vi "TestCloneAPI.vi"() -> ()   [LabVIEW 2018, in "SyncModule.lvlib"]
uses:
  SyncModule.lvlib
  SyncPlugins/SyncPluginBase/Typedefs/clTimedTrigger.ctl
  SyncPlugins/PXI_MultiTrig/Typedefs/clClocks.ctl
  TestInfo.ctl
  <userlib>/NIST/ModuleAdminLib/CloneRegistration/CloneRegistration.lvclass
  <userlib>/NIST/ModuleAdminLib/ModuleAdmin/ModuleAdmin.lvclass/ModuleAdmin.ctl
  <userlib>/NIST/ModuleAdminLib/ModuleAdmin/ModuleAdmin.lvclass
  PublicAPI/Arguments/Broadcasts/clDidInit.ctl
  PublicAPI/Arguments/Requests/clStopArgument.ctl
  <vilib>/Utility/error.llb/DialogType.ctl
  <userlib>/NIST/ModuleAdminLib/ModuleAdmin/Accessors/Read CloneRegRef.vi
  <userlib>/NIST/ModuleAdminLib/ModuleAdmin/Accessors/Write CloneRegRef.vi
  SyncPlugins/SyncPluginBase/SyncPluginBase.lvclass
  SyncPlugins/PXI_MultiTrig/PXI_MultiTrig.lvclass
panel:
  in  "btnSetClkProperties":bool
  in  "ClockProperties":T1[](array[typedef])
  in  "btnClkProperties":bool
  in  "Parameters":string="PXI_Trig2"
  out "Info":string[](array[string])
  in  "btnGetInfo":bool
  in  "Timed Trigger":T2={"TriggerName"="Timed_1", "Time after next UTC Second"=0.1, "Trigger Duration"=0.1, "Edge"=enum."Rising"}
  in  "btnTimedTrig":bool
  in  "btnSoftwareTrig":bool
  in  "btnPref":bool
  out "Locked?":bool
  in  "btnRequestLockStatus":bool
  out "TriggerTime":timestamp format="%^<%.3X\n%x>T"
  in  "btnRequestTriggerTime":bool
  in  "Show Panel":bool=TRUE
  in  "Plugin Type":u16(ring) items=["Local", "NI PXI 6682", "Debug Sync IOP", "6683H class Dyn3", "AbsPhase", "SaveWaveform", "Dyn3 PMU Cal", "HIL_Sync", "Offset Digi Trigger", "PMU Cal Cal"]
  in  "btnLoadPlugin":bool
  out "Path":path
  in  "btnRequestINIPath":bool
  in  "btnRemove":bool
  out "Status Log":string
  out "Active Modules (Array)":string[](array[string])
  in  "btnAdd":bool
  in  "btnStop":bool
  in  "Select Module":i32(ring)=-1 caption="Select Module to send Request" items=["All"=-1, "4140002"=4140002]
  # "Hidden"
  # "Visible"
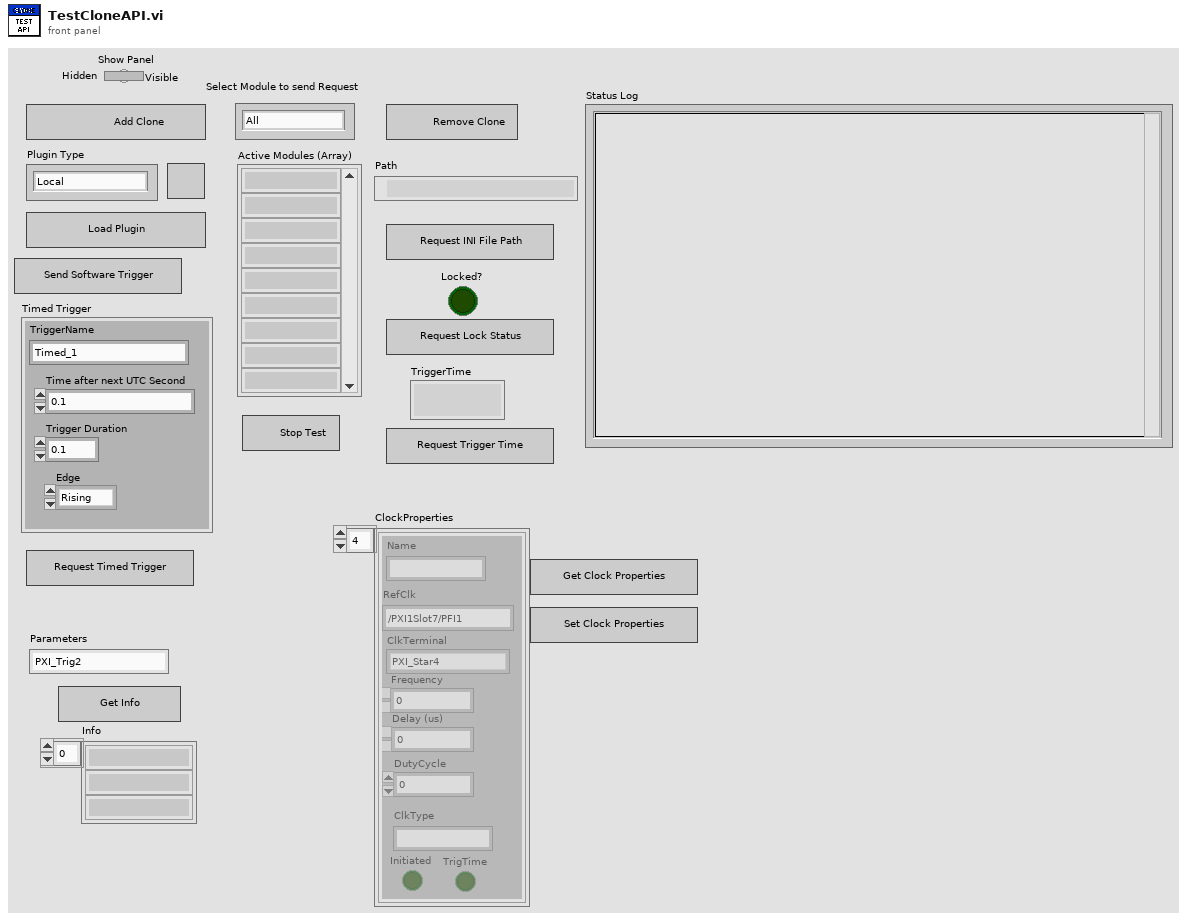
[diagram p1: front panel]
types:
  T1 = typedef "SyncPlugins.lvlib/PXI_MultiTrig.lvclass/clClocks.ctl" = cluster{"Name":string, "RefClk":string, "ClkTerminal":string, "Frequency":dbl, "DutyCycle":dbl, "ClkType":string, "Initiated":bool, "TrigTime":bool, "Delay":dbl}
  T2 = typedef "SyncPlugins.lvlib/SyncPluginBase.lvclass/clTimedTrigger.ctl" = cluster{"TriggerName":string, "Time after next UTC Second":dbl, "Trigger Duration":dbl, "Edge":enum16{"Rising", "Falling"}}
  T3 = typedef "SyncModule.lvlib/TestInfo.ctl" = cluster{"PluginIniFilePaths":path[]}
  T4 = typedef "SyncModule.lvlib/clBroadcastEvents.ctl" = cluster{"DidInit":refnum<user-event>, "StatusUpdate":refnum<user-event>, "ErrorReport":refnum<user-event>, "DidStop":refnum<user-event>, "PathToINI":refnum<user-event>, "TriggerTime":refnum<user-event>, "LockStatus":refnum<user-event>, "Info":refnum<user-event>, "ClockProperties":refnum<user-event>}
  T5 = typedef "SyncModule.lvlib/clDidInit.ctl" = cluster{"Init?":bool, "ModuleAdmin":refnum<class "ModuleAdmin.lvclass">}
  T6 = typedef "SyncModule.lvlib/clStopArgument.ctl" = cluster{"Exit via Stop Module Req?":bool, "Wait for Module to stop?":bool, "ModuleAdmin":refnum<class "ModuleAdmin.lvclass">}
  T7 = typedef "DialogType.ctl" = u16
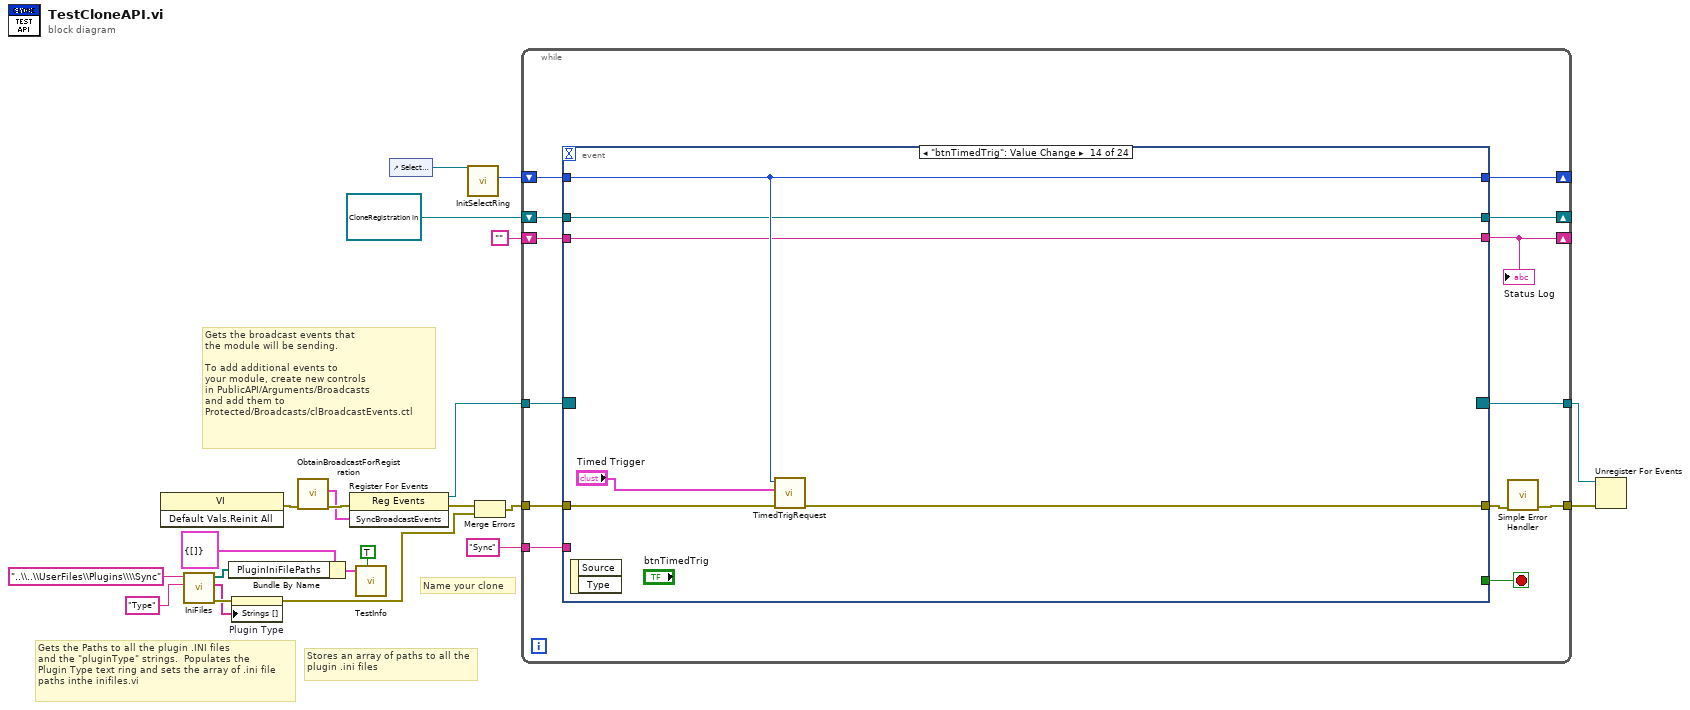
[diagram p0: block diagram]
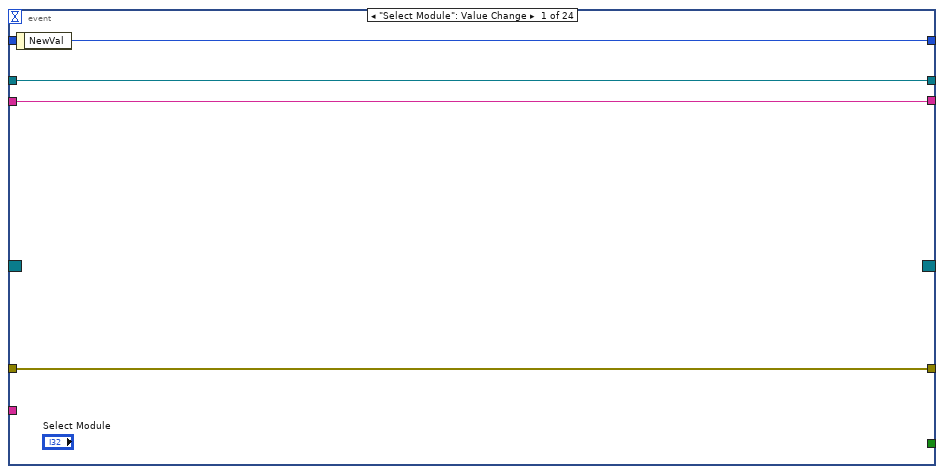
[diagram p2: hidden frame]
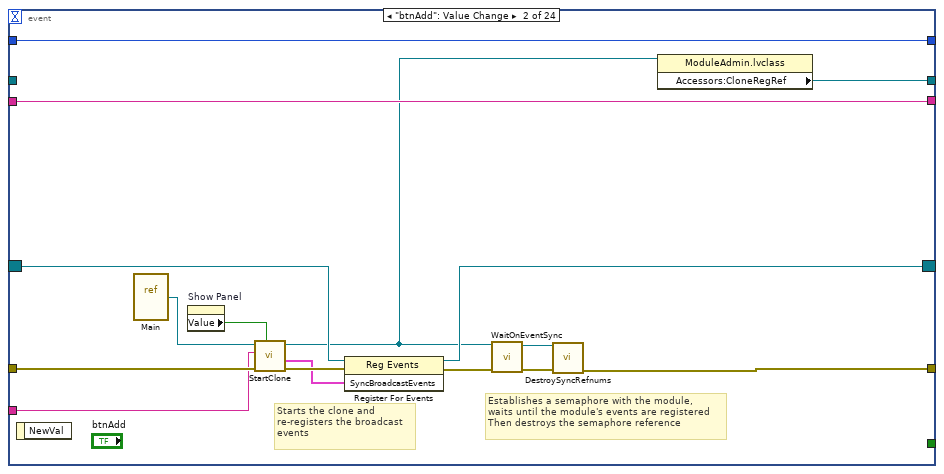
[diagram p3: hidden frame]
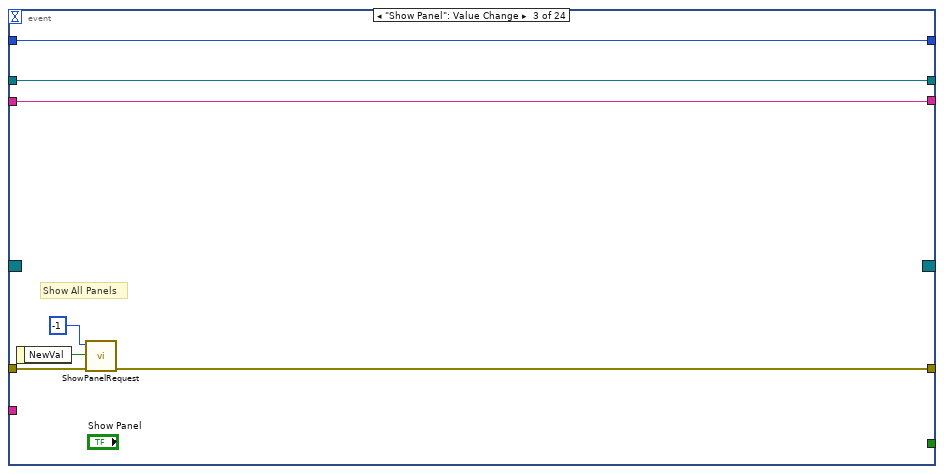
[diagram p4: hidden frame]
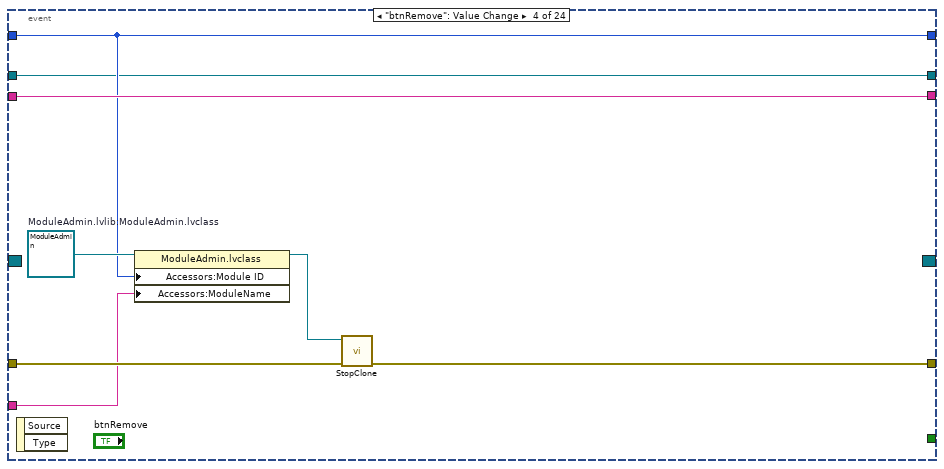
[diagram p5: hidden frame]
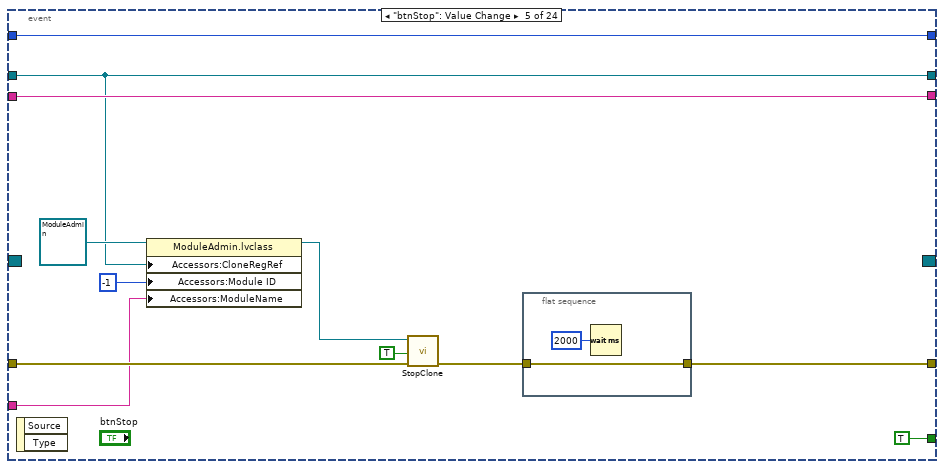
[diagram p6: hidden frame]
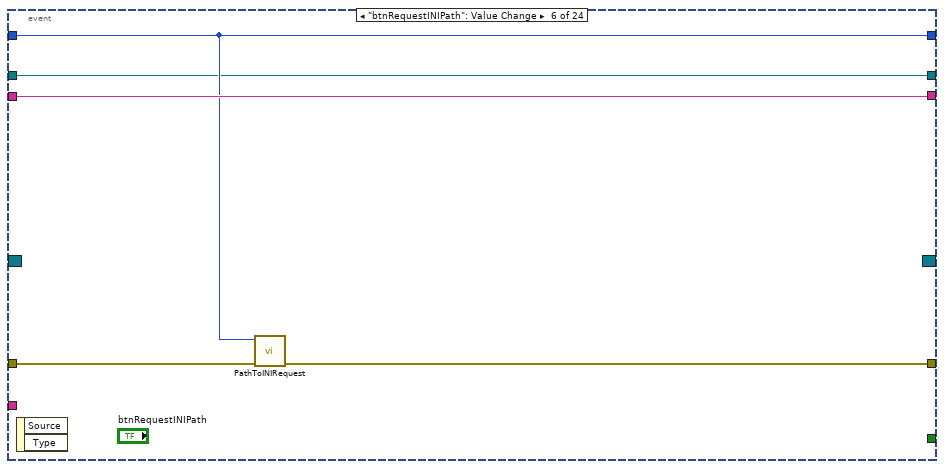
[diagram p7: hidden frame]
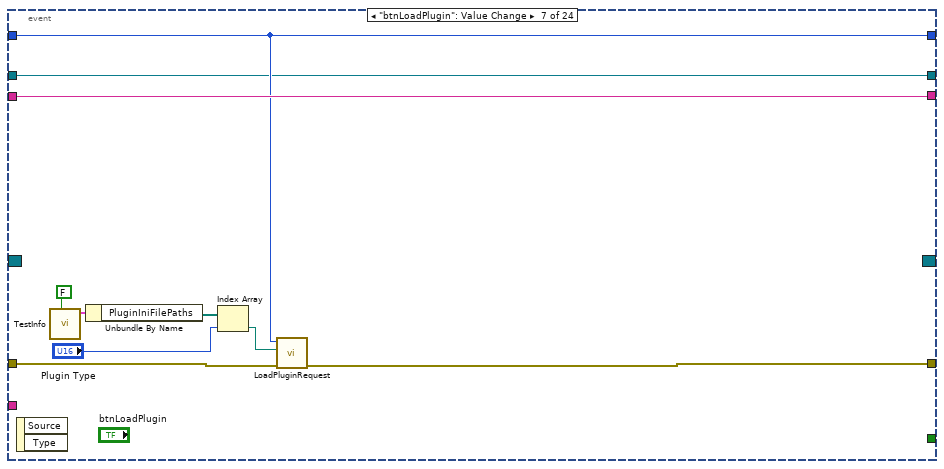
[diagram p8: hidden frame]
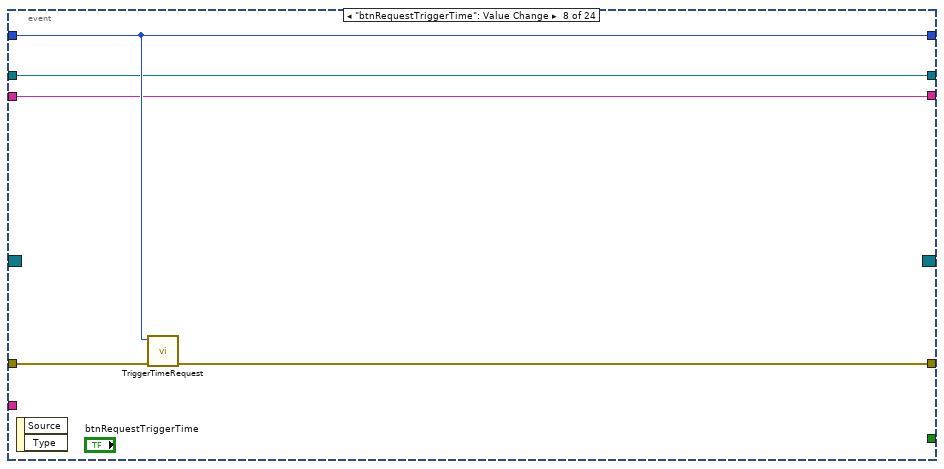
[diagram p9: hidden frame]
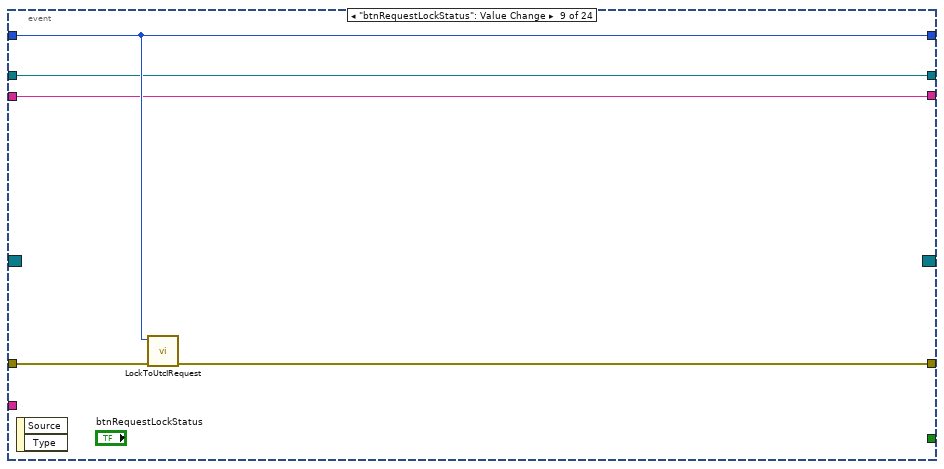
[diagram p10: hidden frame]
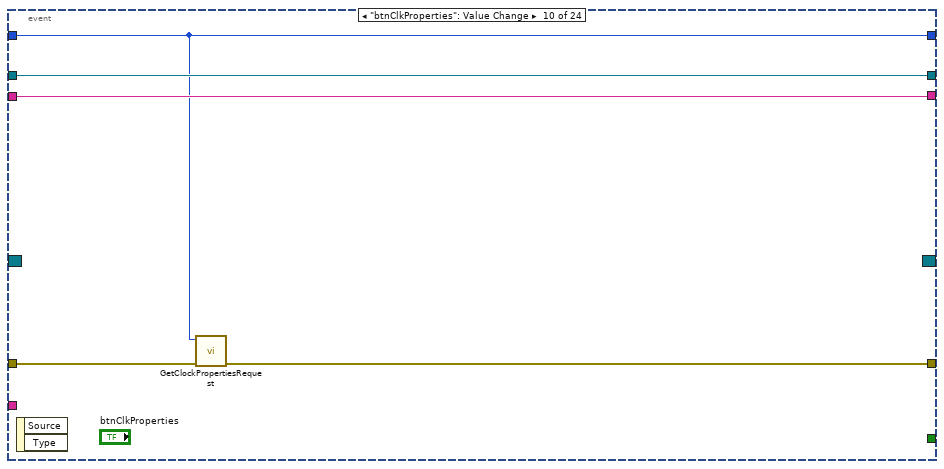
[diagram p11: hidden frame]
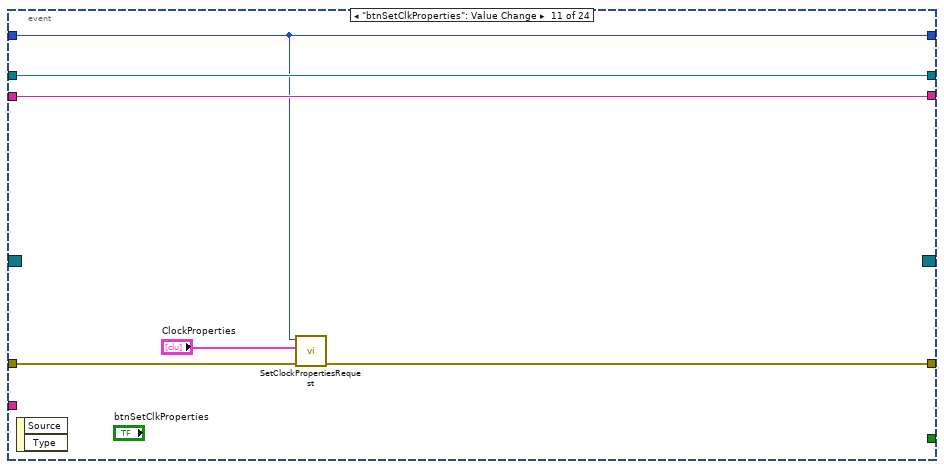
[diagram p12: hidden frame]
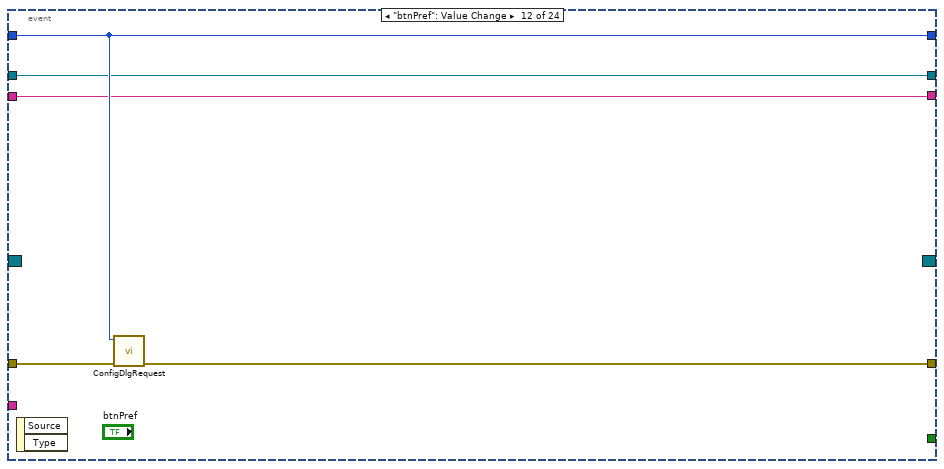
[diagram p13: hidden frame]
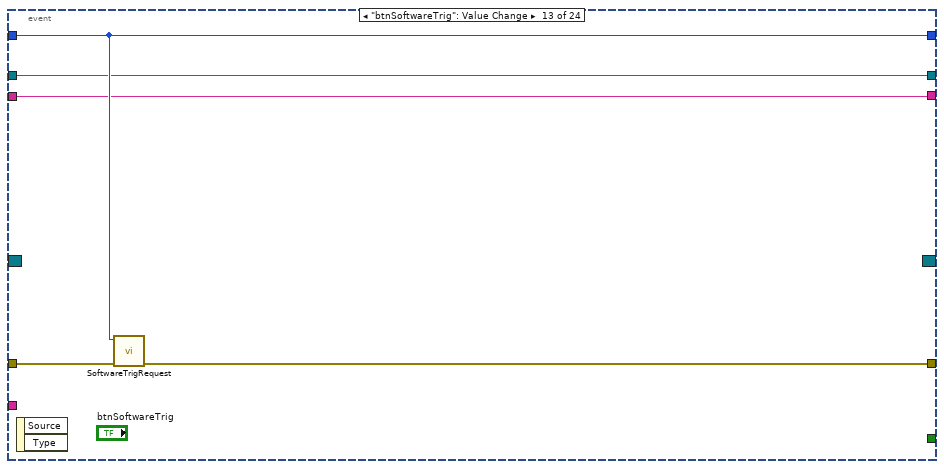
[diagram p14: hidden frame]
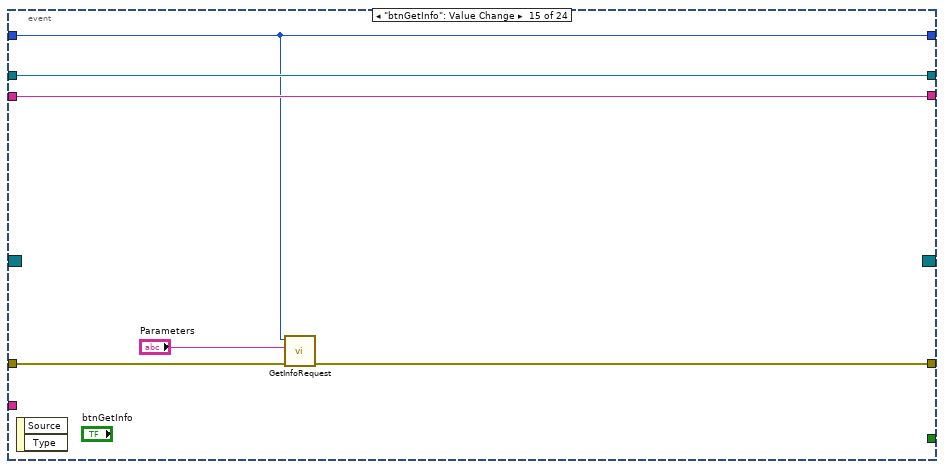
[diagram p15: hidden frame]
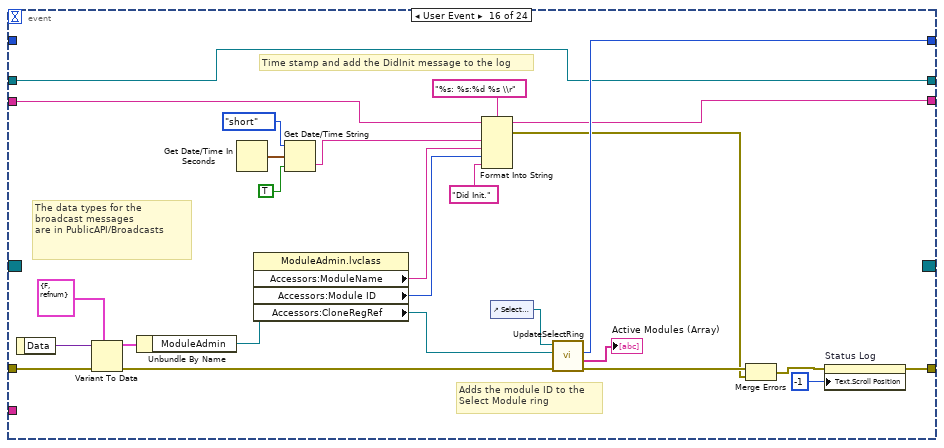
[diagram p16: hidden frame]
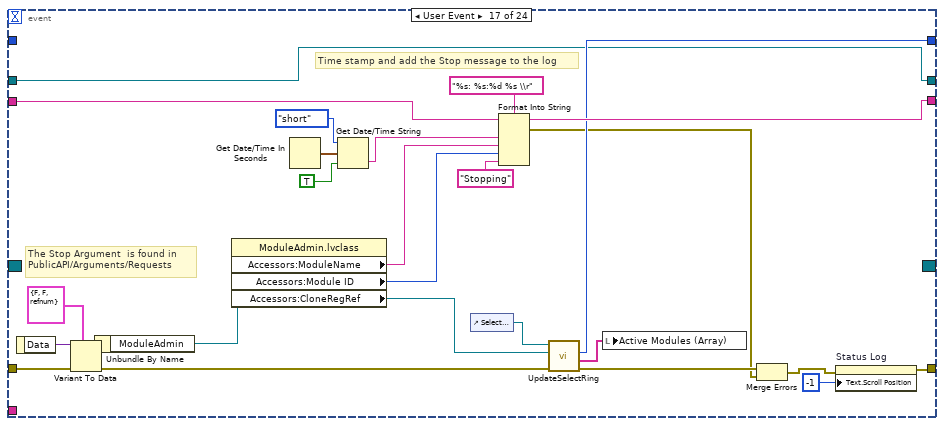
[diagram p17: hidden frame]
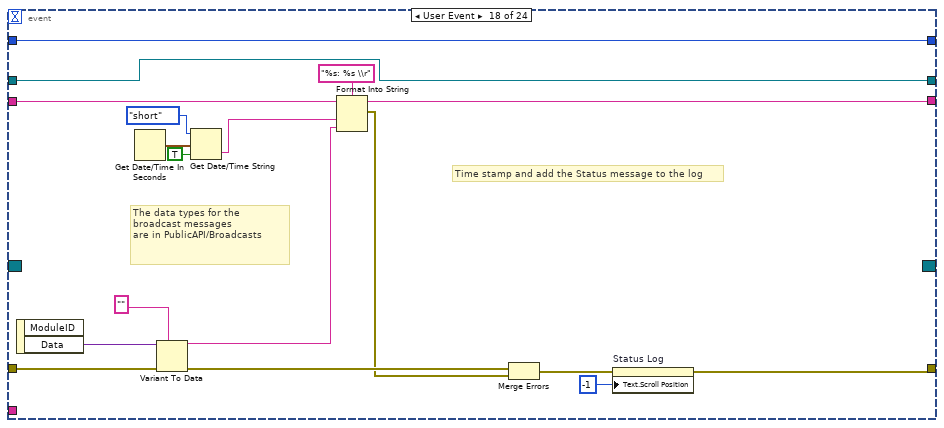
[diagram p18: hidden frame]
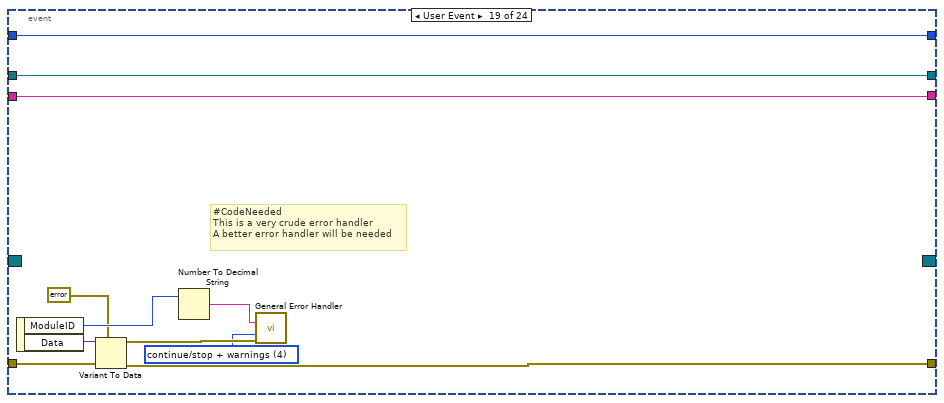
[diagram p19: hidden frame]
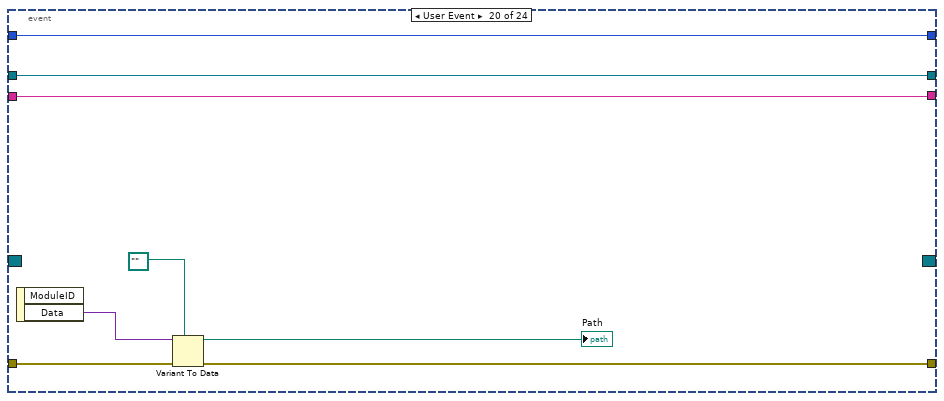
[diagram p20: hidden frame]
diagram:
  # "Stores an array of paths to all the plugin .ini files"
  # "Gets the Paths to all the plugin .INI files\nand the \"pluginType\" strings.  Populates the \nPlugin Type text ring and sets the array of .ini file\npaths inthe inifiles.vi"
  # "Name your clone"
  # "Gets the broadcast events that\nthe module will be sending.\n\nTo add additional events to\nyour module, create new controls\nin PublicAPI/Arguments/Broadcasts\nand add them to\nProtected/Broadcasts/clBroadcastEvents.ctl"
  n1 = invoke class="VI" method="Default Vals.Reinit All"() -> (error out=w20:errorcluster)  [unwired: 3 in, 2 out]
  n2 = call "IniFiles.vi"("iniKey"="Type", "name or relative path"="..\\..\\UserFiles\\Plugins\\\\Sync") -> ("error out"=w13:errorcluster, "Types"=w12:string[], "IniFilePaths"=w11:path[])  [unwired: 7 in]
  n3 = Bundle By Name(cluster=T3 {"PluginIniFilePaths"=[]} ("TestInfo"), "PluginIniFilePaths"=w11) -> (w10:T3)
  n4 = property on="Plugin Type" class="Ring (strict)"(error in=w13, "Strings []"=w12) -> (error out=w7:errorcluster)  [unwired: 1 in, 1 out]
  n5 = call "ObtainBroadcastForRegistration.vi"("error in (no error)"=w20) -> ("error out"=w19:errorcluster, "SyncBroadcastEvents"=w18:T4)  [unwired: 9 in]
  n6 = register-events(error in=w19, w18) -> (reference out=w16:refnum<event-registration>, error out=w17:errorcluster)  [unwired: 1 in]
  n7 = call "TestInfo.vi"("Set (f)"=TRUE, "TestInfo 2"=w10) -> ()  [unwired: 9 in, 1 out]
  n8 = control-ref of="Select Module"() -> (w22:refnum<vi>)
  n9 = call "InitSelectRing.vi"("Ring Refnum"=w22) -> ("Module Ring Value"=w21:i32)  [unwired: 9 in, 1 out]
  n10 = Merge Errors(w17, w7) -> (w8:errorcluster)
  n11 = while {
    shift-right: [w35] -> _
    shift-left: w21 -> [w26]
    tunnel: w8 -> [w33]
    tunnel: w16 -> [w30]
    tunnel: [w31] -> w3
    shift-right: [w29] -> _
    shift-left: "" -> [w28]
    tunnel: "Sync" ("ModuleName") -> [w27]
    tunnel: [w25] -> w2
    shift-right: [w24] -> _
    shift-left: refnum<data-value> refnum ("Accessors:CloneRegRef") -> [w23]
    stop <- w34 stop-if-true
    n12 = event shown="[13] \"btnTimedTrig\": Value Change" {
      selector: w30 -> [_ w47 _ _ _ _ _ _ _ _ _ _ _ _ _ _ _ _ _ _ _ _ _ _]
      dyn-events: [_ w46 _ _ _ _ _ _ _ _ _ _ _ _ _ _ _ _ _ _ _ _ _ _] -> w25
      timeout: _ -> [_ _ _ _ _ _ _ _ _ _ _ _ _ _ _ _ _ _ _ _ _ _ _ _]
      tunnel: w26 -> [_ w55 w58 w66 w82 w88 w96 w103 w108 w111 w116 w124 w129 w135 w138 _ _ w212 w218 w230 w243 w251 w255 w264]
      tunnel: [w39 w55 w58 w66 w82 w88 w96 w103 w108 w111 w116 w124 w129 w135 w138 w163 w181 w212 w218 w230 w243 w251 w255 w264] -> w35
      tunnel: [_ _ _ _ TRUE _ _ _ _ _ _ _ _ _ _ _ _ _ _ _ _ _ _ _] -> w34
      tunnel: w33 -> [w37 w54 w61 w69 w80 w87 w98 w104 w109 w114 w120 w125 w130 w136 w142 w168 w190 w209 w222 w226 w246 w254 w262 w268]
      tunnel: [w37 w48 w59 w68 w71 w86 w97 w101 w106 w110 w119 w121 w126 w132 w137 w144 w170 w197 w221 w225 w233 w252 w258 w267] -> w32
      tunnel: [w38 w44 w57 w70 w78 w89 w99 w102 w107 w113 w118 w123 w128 w134 w140 w156 w187 w206 w217 w231 w240 w250 w257 w266] -> w29
      tunnel: w28 -> [w38 w44 w57 w70 w78 w89 w99 w102 w107 w113 w118 w123 w128 w134 w140 w155 w188 w211 w217 w231 w241 w250 w257 w266]
      tunnel: w27 -> [_ w43 _ w65 w76 _ _ _ _ _ _ _ _ _ _ _ _ _ _ _ _ _ _ _]
      tunnel: [w36 w40 w56 w63 w73 w85 w90 w100 w105 w112 w117 w122 w127 w133 w139 w146 w172 w199 w214 w224 w235 w247 w256 w265] -> w24
      tunnel: w23 -> [w36 _ w56 w63 w73 w85 w90 w100 w105 w112 w117 w122 w127 w133 w139 w146 w172 w199 w214 w224 w235 w247 w256 w265]
      event "Select Module": Value Change {
        n13 = event-data() -> ("NewVal"=w39:i32)  [unwired: 1 in]
      }
      event "btnAdd": Value Change {
        # "Establishes a semaphore with the module,\nwaits until the module's events are registered\nThen destroys the semaphore reference"
        # "Starts the clone and\nre-registers the broadcast \nevents"
        n14 = event-data() -> ()  [unwired: 1 in, 1 out]
        n15 = vi-ref "Main.vi"() -> (w45:refnum<vi>)
        n16 = property on="Show Panel" class="Bool (strict)"() -> ("Value"=w42:bool)  [unwired: 2 in, 2 out]
        n17 = call "StartClone.vi"("ShowPanel? (f)"=w42, "error in (no error)"=w54, "ModuleName"=w43, "VI Refnum"=w45) -> ("error out"=w53:errorcluster, "SyncBroadcastEvents"=w49:T4, "ModuleAdmin"=w41:refnum<class "ModuleAdmin.lvclass">)  [unwired: 5 in]
        n18 = register-events(reference=w47, error in=w53, w49) -> (reference out=w46:refnum<event-registration>, error out=w52:errorcluster)
        n19 = call <userlib>:"WaitOnEventSync.vi"("error in (no error)"=w52, "ModuleAdmin"=w41) -> ("error out"=w51:errorcluster, "ModuleAdmin"=w50:refnum<class "ModuleAdmin.lvclass">)  [unwired: 8 in]
        n20 = call <userlib>:"DestroySyncRefnums.vi"("error in (no error)"=w51, "ModuleAdmin"=w50) -> ("error out"=w48:errorcluster)  [unwired: 9 in]
        n21 = property class="ModuleAdmin.lvclass"(reference=w41) -> ("Accessors:CloneRegRef"=w40:refnum<data-value>)  [unwired: 1 in, 2 out]
      }
      event "Show Panel": Value Change {
        # "Show All Panels"
        n22 = event-data() -> ("NewVal"=w62:bool)  [unwired: 1 in]
        n23 = call "ShowPanelRequest.vi"("error in (no error)"=w61, "ShowPanel?"=w62, "ModuleID"=-1) -> ("error out"=w59:errorcluster)  [unwired: 8 in]
      }
      event "btnRemove": Value Change {
        w67 = refnum<class "ModuleAdmin.lvclass"> refnum  # ModuleAdmin.lvlib:ModuleAdmin.lvclass
        n24 = event-data() -> ()  [unwired: 1 in, 2 out]
        n25 = property class="ModuleAdmin.lvclass"(reference=w67, "Accessors:Module ID"=w66, "Accessors:ModuleName"=w65) -> (reference out=w64:refnum<class "ModuleAdmin.lvclass">)  [unwired: 1 in, 1 out]
        n26 = call "StopClone.vi"("error in (no error)"=w69, "ModuleAdmin"=w64) -> ("error out"=w68:errorcluster)  [unwired: 9 in]
      }
      event "btnStop": Value Change {
        n27 = event-data() -> ()  [unwired: 1 in, 2 out]
        n28 = property class="ModuleAdmin.lvclass"(reference=refnum<class "ModuleAdmin.lvclass"> refnum ("ModuleAdmin.lvlib:ModuleAdmin.lvclass"), "Accessors:CloneRegRef"=w73, "Accessors:Module ID"=-1 ("Module ID"), "Accessors:ModuleName"=w76) -> (reference out=w75:refnum<class "ModuleAdmin.lvclass">)  [unwired: 1 in, 1 out]
        n29 = call "StopClone.vi"("error in (no error)"=w80, "Wait for Module to stop?"=TRUE, "ModuleAdmin"=w75) -> ("error out"=w72:errorcluster)  [unwired: 8 in]
        n30 = flat-sequence {
          tunnel: w72 -> [w83]
          tunnel: [w83] -> w71
          frame #0 {
            n31 = Wait (ms)(milliseconds to wait=u32 2000) -> ()  [unwired: 1 out]
          }
        }
      }
      event "btnRequestINIPath": Value Change {
        n32 = event-data() -> ()  [unwired: 1 in, 2 out]
        n33 = call "PathToINIRequest.vi"("error in (no error)"=w87, "ModuleID"=w88) -> ("error out"=w86:errorcluster)  [unwired: 9 in]
      }
      event "btnLoadPlugin": Value Change {
        n34 = event-data() -> ()  [unwired: 1 in, 2 out]
        n35 = call "TestInfo.vi"("Set (f)"=FALSE) -> ("TestInfo"=w94:T3)  [unwired: 10 in]
        n36 = Unbundle By Name(w94) -> ("PluginIniFilePaths"=w93:path[])
        n37 = Index Array(array=w93, index="Plugin Type") -> (element=w91:path)
        n38 = call "LoadPluginRequest.vi"("error in (no error)"=w98, "PathToPluginINI"=w91, "ModuleID"=w96) -> ("error out"=w97:errorcluster)  [unwired: 8 in]
      }
      event "btnRequestTriggerTime": Value Change {
        n39 = event-data() -> ()  [unwired: 1 in, 2 out]
        n40 = call "TriggerTimeRequest.vi"("error in (no error)"=w104, "ModuleID"=w103) -> ("error out"=w101:errorcluster)  [unwired: 9 in]
      }
      event "btnRequestLockStatus": Value Change {
        n41 = event-data() -> ()  [unwired: 1 in, 2 out]
        n42 = call "LockToUtcIRequest.vi"("error in (no error)"=w109, "ModuleID"=w108) -> ("error out"=w106:errorcluster)  [unwired: 9 in]
      }
      event "btnClkProperties": Value Change {
        n43 = event-data() -> ()  [unwired: 1 in, 2 out]
        n44 = call "GetClockPropertiesRequest.vi"("error in (no error)"=w114, "ModuleID"=w111) -> ("error out"=w110:errorcluster)  [unwired: 9 in]
      }
      event "btnSetClkProperties": Value Change {
        n45 = event-data() -> ()  [unwired: 1 in, 2 out]
        n46 = call "SetClockPropertiesRequest.vi"("error in (no error)"=w120, "ClockProperties"="ClockProperties", "ModuleID"=w116) -> ("error out"=w119:errorcluster)  [unwired: 8 in]
      }
      event "btnPref": Value Change {
        n47 = event-data() -> ()  [unwired: 1 in, 2 out]
        n48 = call "ConfigDlgRequest.vi"("error in (no error)"=w125, "ModuleID"=w124) -> ("error out"=w121:errorcluster)  [unwired: 9 in]
      }
      event "btnSoftwareTrig": Value Change {
        n49 = event-data() -> ()  [unwired: 1 in, 2 out]
        n50 = call "SoftwareTrigRequest.vi"("error in (no error)"=w130, "ModuleID"=w129) -> ("error out"=w126:errorcluster)  [unwired: 9 in]
      }
      event "btnTimedTrig": Value Change {
        n51 = event-data() -> ()  [unwired: 1 in, 2 out]
        n52 = call "TimedTrigRequest.vi"("error in (no error)"=w136, "Time after next UTC Second"="Timed Trigger", "ModuleID"=w135) -> ("error out"=w132:errorcluster)  [unwired: 8 in]
      }
      event "btnGetInfo": Value Change {
        n53 = event-data() -> ()  [unwired: 1 in, 2 out]
        n54 = call "GetInfoRequest.vi"("error in (no error)"=w142, "Parameters"="Parameters", "ModuleID"=w138) -> ("error out"=w137:errorcluster)  [unwired: 8 in]
      }
      event User Event {
        # "Adds the module ID to the \nSelect Module ring"
        # "Time stamp and add the DidInit message to the log"
        # "The data types for the broadcast messages\nare in PublicAPI/Broadcasts"
        n55 = event-data() -> ("Data"=w167:variant)  [unwired: 1 in]
        n56 = Variant To Data(error in=w168, type=T5 {"Init?"=FALSE, "ModuleAdmin"=refnum} ("clDidInit"), Variant=w167) -> (data=w160:T5, error out=w165:errorcluster)
        n57 = Unbundle By Name(w160) -> ("ModuleAdmin"=w151:refnum<class "ModuleAdmin.lvclass">)
        n58 = Get Date/Time In Seconds() -> (seconds since 1Jan1904=w158:timestamp)
        n59 = property class="ModuleAdmin.lvclass"(reference=w151) -> ("Accessors:ModuleName"=w149:string, "Accessors:Module ID"=w148:i32, "Accessors:CloneRegRef"=w147:refnum<data-value>)  [unwired: 1 in, 2 out]
        n60 = Get Date/Time String(date format (0)=enum16{"short", "long", "abbreviated"}."short", seconds (now)=w158, want seconds? (F)=TRUE) -> (time string=w161:string)  [unwired: 1 out]
        n61 = Format Into String(format string="%s: %s:%d %s \\r", initial string=w155, w161, w149, w148, "Did Init.") -> (resulting string=w156:string, error out=w153:errorcluster)  [unwired: 1 in]
        n62 = control-ref of="Select Module"() -> (w164:refnum<vi>)
        n63 = call "UpdateSelectRing.vi"("error in (no error)"=w165, "CloneRegRef"=w147, "Ring Refnum"=w164) -> ("error out"=w154:errorcluster, "ActiveModules"=→"Active Modules (Array)":string[], "Module Ring Value"=w163:i32)  [unwired: 6 in]
        n64 = Merge Errors(w154, w153) -> (w143:errorcluster)
        n65 = property on="Status Log" class="Str"(error in=w143, "Text.Scroll Position"=-1) -> (error out=w144:errorcluster)  [unwired: 1 in, 1 out]
      }
      event User Event {
        # "Time stamp and add the Stop message to the log"
        # "The Stop Argument  is found in\nPublicAPI/Arguments/Requests"
        n66 = event-data() -> ("Data"=w189:variant)  [unwired: 1 in]
        n67 = Variant To Data(error in=w190, type=T6 {"Exit via Stop Module Req?"=FALSE, "Wait for Module to stop?"=FALSE, "ModuleAdmin"=refnum} ("Stop Argument"), Variant=w189) -> (data=w185:T6, error out=w184:errorcluster)
        n68 = Unbundle By Name(w185) -> ("ModuleAdmin"=w177:refnum<class "ModuleAdmin.lvclass">)
        n69 = property class="ModuleAdmin.lvclass"(reference=w177) -> ("Accessors:ModuleName"=w175:string, "Accessors:Module ID"=w174:i32, "Accessors:CloneRegRef"=w173:refnum<data-value>)  [unwired: 1 in, 2 out]
        n70 = Get Date/Time In Seconds() -> (seconds since 1Jan1904=w192:timestamp)
        n71 = Get Date/Time String(date format (0)=enum16{"short", "long", "abbreviated"}."short", seconds (now)=w192, want seconds? (F)=TRUE) -> (time string=w194:string)  [unwired: 1 out]
        n72 = control-ref of="Select Module"() -> (w183:refnum<vi>)
        n73 = Format Into String(format string="%s: %s:%d %s \\r", initial string=w188, w194, w175, w174, "Stopping") -> (resulting string=w187:string, error out=w179:errorcluster)  [unwired: 1 in]
        n74 = call "UpdateSelectRing.vi"("error in (no error)"=w184, "CloneRegRef"=w173, "Ring Refnum"=w183) -> ("error out"=w180:errorcluster, "ActiveModules"=w182:string[], "Module Ring Value"=w181:i32)  [unwired: 6 in]
        n75 = local write "Active Modules (Array)"(w182) -> ()
        n76 = Merge Errors(w180, w179) -> (w169:errorcluster)
        n77 = property on="Status Log" class="Str"(error in=w169, "Text.Scroll Position"=-1) -> (error out=w170:errorcluster)  [unwired: 1 in, 1 out]
      }
      event User Event {
        # "Time stamp and add the Status message to the log"
        # "The data types for the broadcast messages\nare in PublicAPI/Broadcasts"
        n78 = event-data() -> ("Data"=w208:variant)  [unwired: 1 in, 1 out]
        n79 = Get Date/Time In Seconds() -> (seconds since 1Jan1904=w207:timestamp)
        n80 = Variant To Data(error in=w209, type="", Variant=w208) -> (data=w195:string, error out=w205:errorcluster)
        n81 = Get Date/Time String(date format (0)=enum16{"short", "long", "abbreviated"}."short", seconds (now)=w207, want seconds? (F)=TRUE) -> (time string=w201:string)  [unwired: 1 out]
        n82 = Format Into String(format string="%s: %s \\r", initial string=w211, w201, w195) -> (resulting string=w206:string, error out=w204:errorcluster)  [unwired: 1 in]
        n83 = Merge Errors(w205, w204) -> (w198:errorcluster)
        n84 = property on="Status Log" class="Str"(error in=w198, "Text.Scroll Position"=-1) -> (error out=w197:errorcluster)  [unwired: 1 in, 1 out]
      }
      event User Event {
        w213 = T7 4 items=["no dialog", "OK message", "continue or stop message", "OK message + warnings", "continue/stop + warnings"] ("type of dialog (OK msg:1)")
        # "#CodeNeeded\nThis is a very crude error handler\nA better error handler will be needed"
        n85 = event-data() -> ("ModuleID"=w220:i32, "Data"=w223:variant)  [unwired: 1 in]
        n86 = Variant To Data(error in=w222, type=errorcluster {"status"=FALSE, "code"=0, "source"=""} ("error constant"), Variant=w223) -> (data=w215:errorcluster, error out=w221:errorcluster)
        n87 = Number To Decimal String(number=w220) -> (decimal integer string=w219:string)  [unwired: 1 in]
        n88 = call <vilib>:"General Error Handler.vi"("[error source] (\" \")"=w219, "type of dialog (OK msg:1)"=w213, "error in (no error)"=w215) -> ()  [unwired: 8 in, 5 out]
      }
      event User Event {
        n89 = event-data() -> ("Data"=w228:variant)  [unwired: 1 in, 1 out]
        n90 = Variant To Data(error in=w226, type=path "" ("Path"), Variant=w228) -> (data=→"Path":path, error out=w225:errorcluster)
      }
      event User Event {
        n91 = event-data() -> ("Data"=w245:variant)  [unwired: 1 in, 1 out]
        n92 = Variant To Data(error in=w246, type=0.0, Variant=w245) -> (data=w236:dbl, error out=w239:errorcluster)
        n93 = To Time Stamp(1:w236) -> (0:→"TriggerTime":timestamp)
        n94 = Format Into String(format string="Trigger Time: %f \\r", initial string=w241, w236) -> (resulting string=w240:string, error out=w238:errorcluster)  [unwired: 1 in]
        n95 = Merge Errors(w238, w239) -> (w232:errorcluster)
        n96 = property on="Status Log" class="Str"(error in=w232, "Text.Scroll Position"=-1) -> (error out=w233:errorcluster)  [unwired: 1 in, 1 out]
      }
      event User Event {
        n97 = event-data() -> ("Data"=w253:variant)  [unwired: 1 in, 1 out]
        n98 = Variant To Data(error in=w254, type=TRUE, Variant=w253) -> (data=→"Locked?":bool, error out=w252:errorcluster)
      }
      event User Event {
        n99 = event-data() -> ("Data"=w261:variant)  [unwired: 1 in, 1 out]
        n100 = Variant To Data(error in=w262, type=string[] [], Variant=w261) -> (data=→"Info":string[], error out=w258:errorcluster)
      }
      event User Event {
        n101 = event-data() -> ("Data"=w270:variant)  [unwired: 1 in, 1 out]
        n102 = Variant To Data(error in=w268, type=T1[] [], Variant=w270) -> (data=w263:T1[], error out=w267:errorcluster)
        n103 = local write "ClockProperties"(w263) -> ()
      }
    }
    "Status Log" <- w29
    n104 = call <vilib>:"Simple Error Handler.vi"("error in (no error)"=w32) -> ("error out"=w31:errorcluster)  [unwired: 4 in, 4 out]
  }
  n105 = Unregister For Events(event registration refnum=w2, error in=w3) -> ()  [unwired: 1 out]
